vi "Configure.vi"(7 "Setpoint Deceleration":u32, 8 "error in (no error)":errorcluster, 9 "Setpoint Acceleration":u32, 10 "Setpoint Velocity":u32, 11 "MotorDrive in":refnum<class "MotorDrive.lvclass">) -> (0 "error out":errorcluster, 3 "MotorDrive out":refnum<class "MotorDrive.lvclass">)   [LabVIEW 2016, in "MotorDrive.lvclass"]
uses:
  MotorDrive.lvclass
  MotorDrive.lvclass/MotorDrive.ctl
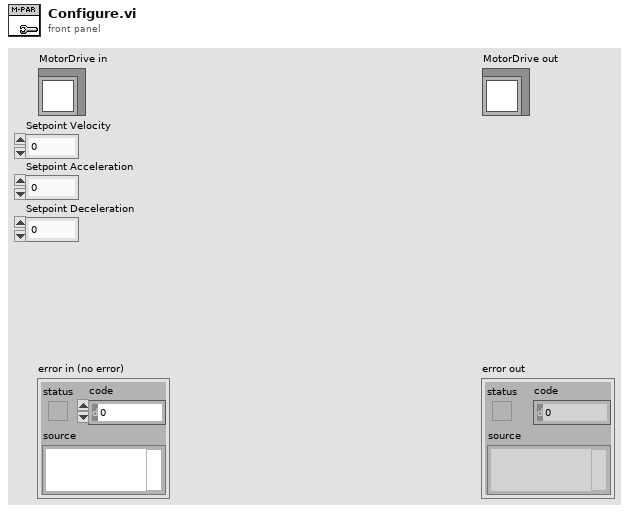
[diagram p1: front panel]
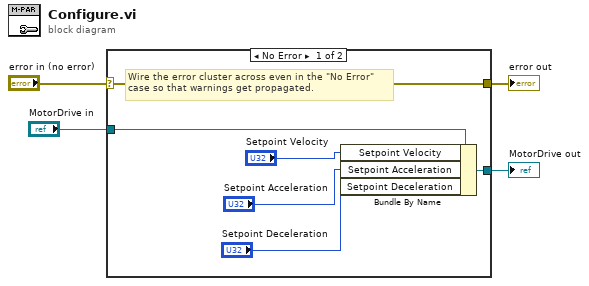
[diagram p0: block diagram]
diagram:
  n1 = case shown="No Error" "error in (no error)" {
    selector: "error in (no error)" -> [w9 w12]
    tunnel: [w9 w12] -> w3
    tunnel: [w8 w11] -> w1
    tunnel: "MotorDrive in" -> [w10 w11]
    frame No Error {
      # "Wire the error cluster across even in the \"No Error\"\ncase so that warnings get propagated."
      n2 = Bundle By Name(cluster=w10, "Setpoint Velocity"="Setpoint Velocity", "Setpoint Acceleration"="Setpoint Acceleration", "Setpoint Deceleration"="Setpoint Deceleration") -> (w8:refnum<class "MotorDrive.lvclass">)
    }
    frame Error {
    }
  }
  "error out" <- w3
  "MotorDrive out" <- w1
